vi "Scan Setup.vi"(8 "error in (no error)":errorcluster, 11 "Pulse Gen Basic Scan in":refnum<class "Pulse Gen Basic Scan.lvclass">) -> (0 "error out":errorcluster, 3 "Pulse Gen Basic Scan out":refnum<class "Pulse Gen Basic Scan.lvclass">)   [LabVIEW 2009, in "Pulse Gen Basic Scan.lvclass"]
doc: "Configure the Instrument based on the class member fields. This step comes after the user has closed the \"Scan Setup\" window and before the actual scan -- so instruments are configured with the user's specified settings."
uses:
  Pulse Gen Basic Scan.lvclass
  Scanner/Scanner.lvclass
  Instruments/Utility Classes/Scannable/Scannable.lvclass
  Pulse Gen Basic Scan.lvclass/Pulse Gen Basic Scan.ctl
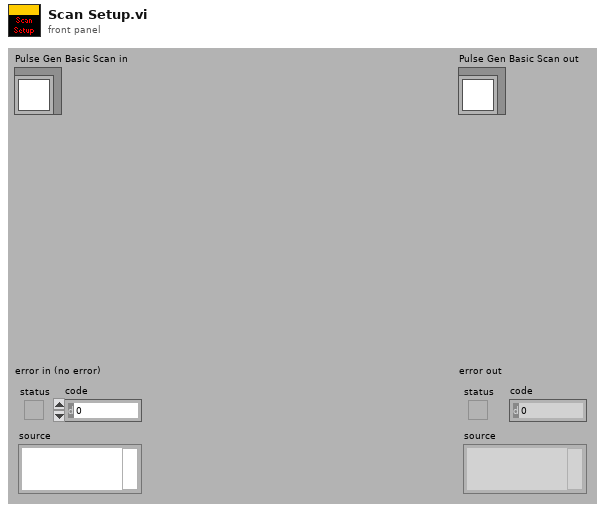
[diagram p1: front panel]
types:
  T1 = enum16{"Internal Oscillator", "Internal PLL", "External Clock "}
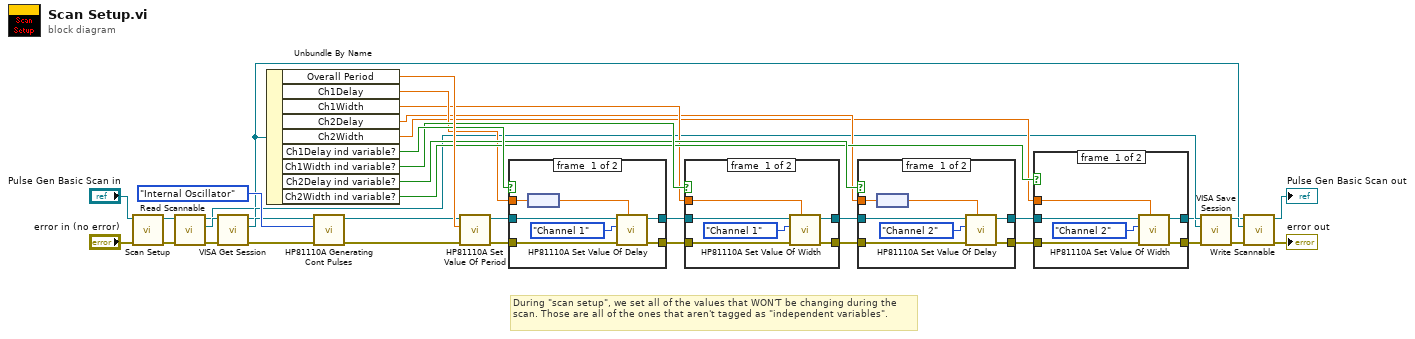
[diagram p0: block diagram]
diagram:
  # "During \"scan setup\", we set all of the values that WON'T be changing during the scan. Those are all of the ones that aren't tagged as \"independent variables\"."
  n1 = call-parent "Scan Setup.vi"("error in (no error)"="error in (no error)", "Scanner in"="Pulse Gen Basic Scan in") -> ("error out"=w13:errorcluster, "Scanner out"=w14:refnum<class "Pulse Gen Basic Scan.lvclass">)  [unwired: 8 in]
  n2 = call-dynamic "Read Scannable.vi"("error in (no error)"=w13, "Scanner.lvclass in"=w14) -> ("error out"=w10:errorcluster, "Scannable.lvclass"=w12:refnum<class "Scannable.lvclass">, "Scanner.lvclass out"=w3:refnum<class "Pulse Gen Basic Scan.lvclass">)  [unwired: 7 out]
  n3 = call-dynamic "VISA Get Session.vi"("error in (no error)"=w10, "Instrument.lvclass in"=w12) -> ("error out"=w9:errorcluster, "VISA Resource Name"=w11:refnum<visa-resource-name>, "Instrument.lvclass out"=w8:refnum<class "Scannable.lvclass">)  [unwired: 7 out]
  n4 = Unbundle By Name(w3) -> ("Overall Period"=w33:dbl[unit], "Ch1Delay"=w18:dbl[unit], "Ch1Width"=w17:dbl[unit], "Ch2Delay"=w16:dbl[unit], "Ch2Width"=w15:dbl[unit], "Ch1Delay ind variable?"=w30:bool, "Ch1Width ind variable?"=w29:bool, "Ch2Delay ind variable?"=w28:bool, "Ch2Width ind variable?"=w27:bool)
  n5 = call "HP81110A Generating Cont Pulses.vi"("error in (no error)"=w9, "Period Source (0:Internal)"=T1."Internal Oscillator", "VISA session"=w11) -> ("error out"=w31:errorcluster, "dup VISA session"=w32:refnum<visa-resource-name>)  [unwired: 7 in]
  n6 = call "HP81110A Set Value Of Period.vi"("error in (no error)"=w31, "Period Value"=w33, "VISA session"=w32) -> ("error out"=w22:errorcluster, "dup VISA session"=w26:refnum<visa-resource-name>)  [unwired: 7 in]
  n7 = case shown="False" w30 {
    tunnel: w26 -> [w43 w45]
    tunnel: [w42 w45] -> w25
    tunnel: w22 -> [w41 w44]
    tunnel: [w40 w44] -> w21
    tunnel: w18 -> [w38 _]
    frame #0 {
      n8 = node(w38) -> (w37:dbl)
      n9 = call "HP81110A Set Value Of Delay.vi"("Delay Value (0.0)"=w37, "error in (no error)"=w41, "Channel (1:Channel 1)"=enum16{"Channel All ", "Channel 1", "Channel 2"}."Channel 1", "VISA session"=w43) -> ("error out"=w40:errorcluster, "dup VISA session"=w42:refnum<visa-resource-name>)  [unwired: 6 in]
    }
    frame #1 {
    }
  }
  n10 = case shown="False" w29 {
    tunnel: w25 -> [w51 w53]
    tunnel: [w50 w53] -> w24
    tunnel: w21 -> [w49 w52]
    tunnel: [w48 w52] -> w20
    tunnel: w17 -> [w46 _]
    frame #0 {
      n11 = call "HP81110A Set Value Of Width.vi"("Width Value (100.0E-9)"=w46, "error in (no error)"=w49, "Channel (1:Channel 1)"=enum16{"Channel All ", "Channel 1", "Channel 2"}."Channel 1", "VISA session"=w51) -> ("error out"=w48:errorcluster, "dup VISA session"=w50:refnum<visa-resource-name>)  [unwired: 6 in]
    }
    frame #1 {
    }
  }
  n12 = case shown="False" w28 {
    tunnel: w24 -> [w60 w62]
    tunnel: [w59 w62] -> w23
    tunnel: w20 -> [w58 w61]
    tunnel: [w57 w61] -> w19
    tunnel: w16 -> [w55 _]
    frame #0 {
      n13 = node(w55) -> (w54:dbl)
      n14 = call "HP81110A Set Value Of Delay.vi"("Delay Value (0.0)"=w54, "error in (no error)"=w58, "Channel (1:Channel 1)"=enum16{"Channel All ", "Channel 1", "Channel 2"}."Channel 2", "VISA session"=w60) -> ("error out"=w57:errorcluster, "dup VISA session"=w59:refnum<visa-resource-name>)  [unwired: 6 in]
    }
    frame #1 {
    }
  }
  n15 = case shown="False" w27 {
    tunnel: w23 -> [w68 w69]
    tunnel: w19 -> [w67 w70]
    tunnel: [w66 w70] -> w5
    tunnel: w15 -> [w64 _]
    tunnel: [w63 w69] -> w7
    frame #0 {
      n16 = call "HP81110A Set Value Of Width.vi"("Width Value (100.0E-9)"=w64, "error in (no error)"=w67, "Channel (1:Channel 1)"=enum16{"Channel All ", "Channel 1", "Channel 2"}."Channel 2", "VISA session"=w68) -> ("error out"=w66:errorcluster, "dup VISA session"=w63:refnum<visa-resource-name>)  [unwired: 6 in]
    }
    frame #1 {
    }
  }
  n17 = call-dynamic "VISA Save Session.vi"("error in (no error)"=w5, "VISA Resource Name"=w7, "Instrument.lvclass in"=w8) -> ("error out"=w6:errorcluster, "Instrument.lvclass out"=w4:refnum<class "Scannable.lvclass">)  [unwired: 7 out]
  n18 = call-dynamic "Write Scannable.vi"("error in (no error)"=w6, "Scannable.lvclass"=w4, "Scanner.lvclass in"=w3) -> ("error out"=→"error out":errorcluster, "Scanner.lvclass out"=→"Pulse Gen Basic Scan out":refnum<class "Pulse Gen Basic Scan.lvclass">)  [unwired: 7 out]
